vi "Create Channel Headers.vi"(8 "Error In":errorcluster, 9 "Channel Names":string[](array[string]), 11 "File Refnum In":refnum<file>) -> (0 "Error Out":errorcluster, 3 "File Refnum Out":refnum<file>)   [LabVIEW 2014]
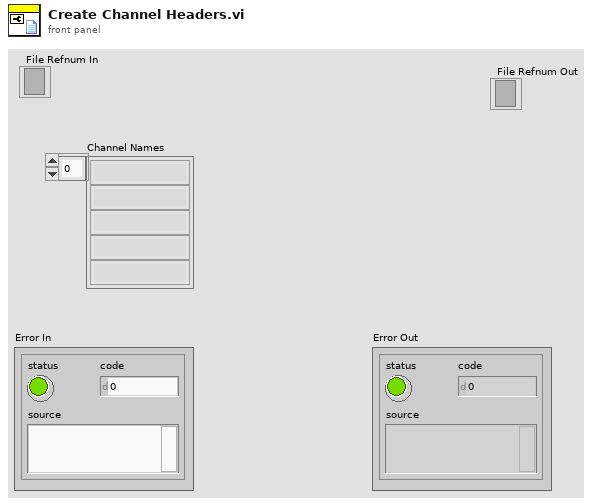
[diagram p1: front panel]
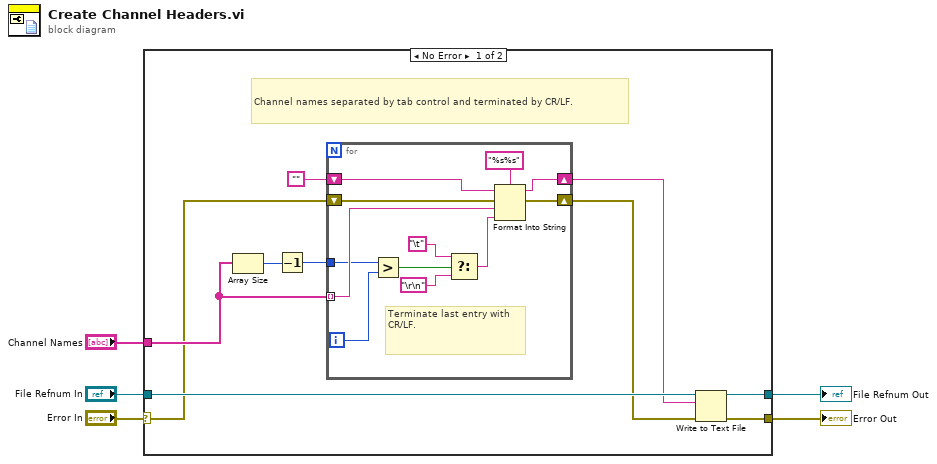
[diagram p0: block diagram]
diagram:
  n1 = case shown="No Error" "Error In" {
    selector: "Error In" -> [w7 w28]
    tunnel: [w13 w28] -> w3
    tunnel: "File Refnum In" -> [w15 w29]
    tunnel: [w14 w29] -> w4
    tunnel: "Channel Names" -> [w10 _]
    frame No Error {
      # "Channel names separated by tab control and terminated by CR/LF."
      n2 = Array Size(array=w10) -> (size(s)=w12:i32)
      n3 = Decrement(x=w12) -> (x-1=w11:i32)
      n4 = for {
        shift-right: [w26] -> w8
        shift-left: "" -> [w27]
        tunnel: w10 -> [w25] mode=indexing
        shift-right: [w23] -> w6
        shift-left: w7 -> [w24]
        tunnel: w11 -> [w18]
        i -> [w17]
        # "Terminate last entry with CR/LF."
        n5 = Greater?(x=w18, y=w17) -> (0:w16:bool)
        n6 = Select(t="\t", s=w16, f="\r\n") -> (s? t:f=w21:string)
        n7 = Format Into String(format string="%s%s", initial string=w27, error in=w24, w25, w21) -> (resulting string=w26:string, error out=w23:errorcluster)
      }
      n8 = Write to Text File(file (use dialog)=w15, text=w8, error in=w6) -> (refnum out=w14:refnum<file>, error out=w13:errorcluster)  [unwired: 1 in, 1 out]
    }
    frame Error {
    }
  }
  "File Refnum Out" <- w4
  "Error Out" <- w3
